vi "ErrorMngmt_Read.vi"() -> ()   [LabVIEW 2015]
panel:
  out "Target Disconnected?":bool
  out "data out":bool
  out "error out 2":errorcluster
  out "error out":errorcluster
  in  "stop":bool
  out "Errors":string[](array[string])
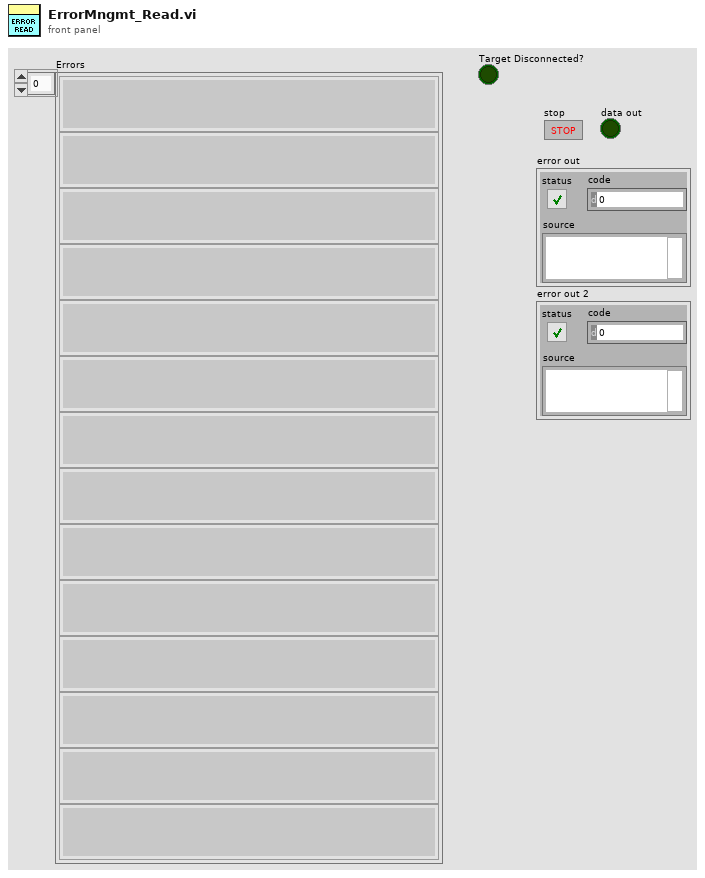
[diagram p1: front panel]
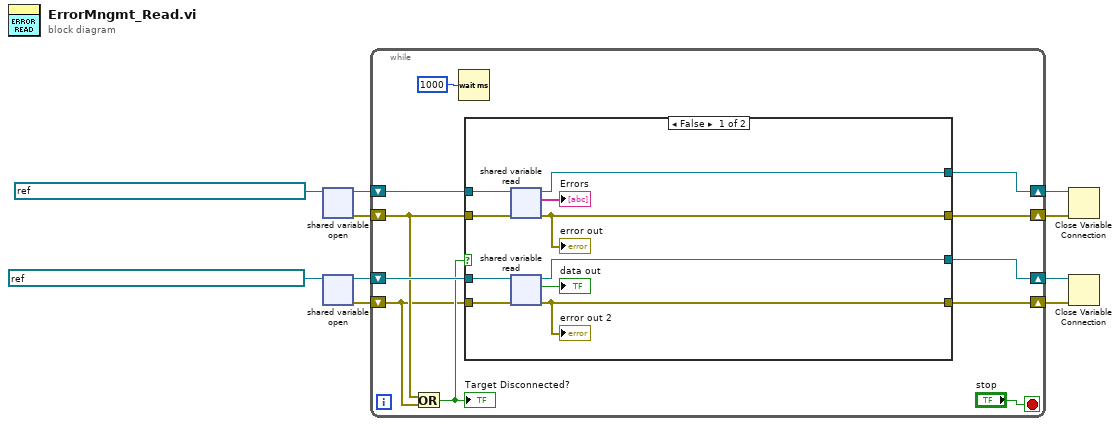
[diagram p0: block diagram]
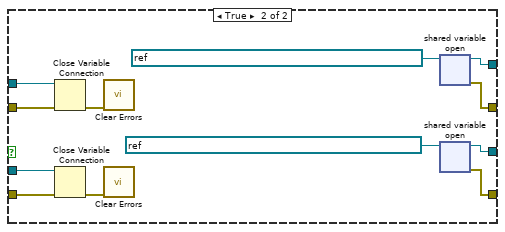
[diagram p2: hidden frame]
diagram:
  n1 = shared-variable-open(refnum<k21> "ni.var.psp://NI-myRIO-1900-NIPH/Monitoring/Errors" ("shared variable refnum in")) -> (w9:refnum<k21>, w8:errorcluster)  [unwired: 1 in]
  n2 = shared-variable-open(refnum<k21> "ni.var.psp://NI-myRIO-1900-NIPH/WebResources/Key" ("shared variable refnum in")) -> (w5:refnum<k21>, w3:errorcluster)  [unwired: 1 in]
  n3 = while {
    shift-right: [w20] -> w7
    shift-left: w9 -> [w21]
    shift-right: [w19] -> w6
    shift-left: w8 -> [w13]
    shift-right: [w15] -> w2
    shift-left: w3 -> [w12]
    shift-right: [w16] -> w4
    shift-left: w5 -> [w17]
    stop <- "stop" stop-if-true
    n4 = Or(x=w13, y=w12) -> (x .or. y?=w14:bool)
    "Target Disconnected?" <- w14
    n5 = Wait (ms)(milliseconds to wait=u32 1000) -> ()  [unwired: 1 out]
    n6 = case shown="False" w14 {
      tunnel: w21 -> [w31 w43]
      tunnel: w13 -> [w30 w42]
      tunnel: [w28 w37] -> w20
      tunnel: [w27 w36] -> w19
      tunnel: w17 -> [w26 w41]
      tunnel: [w25 w35] -> w16
      tunnel: w12 -> [w24 w40]
      tunnel: [w23 w34] -> w15
      frame False {
        n7 = shared-variable-read(w31, w30) -> (w28:refnum<k21>, w27:errorcluster, →"Errors":string[])
        "error out" <- w27
        n8 = shared-variable-read(w26, w24) -> (w25:refnum<k21>, w23:errorcluster, →"data out":bool)
        "error out 2" <- w23
      }
      frame True {
        n9 = Close Variable Connection(8:w42, 11:w43) -> (0:w33:errorcluster)
        n10 = Close Variable Connection(8:w40, 11:w41) -> (0:w32:errorcluster)
        n11 = call <vilib>:"Clear Errors.vi"("error in (no error)"=w33) -> ()  [unwired: 5 in, 2 out]
        n12 = call <vilib>:"Clear Errors.vi"("error in (no error)"=w32) -> ()  [unwired: 5 in, 2 out]
        n13 = shared-variable-open(refnum<k21> "ni.var.psp://NI-myRIO-1900-NIPH/Monitoring/Errors" ("shared variable refnum in")) -> (w37:refnum<k21>, w36:errorcluster)  [unwired: 1 in]
        n14 = shared-variable-open(refnum<k21> "ni.var.psp://NI-myRIO-1900-NIPH/WebResources/Key" ("shared variable refnum in")) -> (w35:refnum<k21>, w34:errorcluster)  [unwired: 1 in]
      }
    }
  }
  n15 = Close Variable Connection(8:w6, 11:w7) -> ()  [unwired: 1 out]
  n16 = Close Variable Connection(8:w2, 11:w4) -> ()  [unwired: 1 out]
